vi "Filter Aliases.vi"(8 "error in (no error)":errorcluster, 9 "INI.Client.Type":T1, 10 "Alias.FolderPath":string, 11 "Aliases":string[](array[string])) -> (0 "error out":errorcluster, 2 "Tag.Names":string[](array[string]), 3 "Aliases":string[](array[string]))   [LabVIEW 2019, in "Data Publishing Service.lvlib"]
uses:
  Data Publishing Service.lvlib
  Types/ClientType.ctl
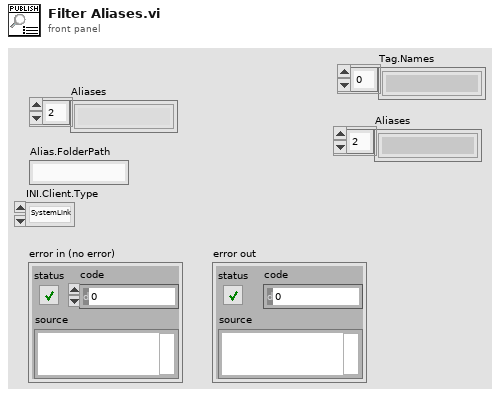
[diagram p1: front panel]
types:
  T1 = typedef "Data Publishing Service.lvlib/ClientType.ctl" = enum16{"SystemLink", "DSC"}
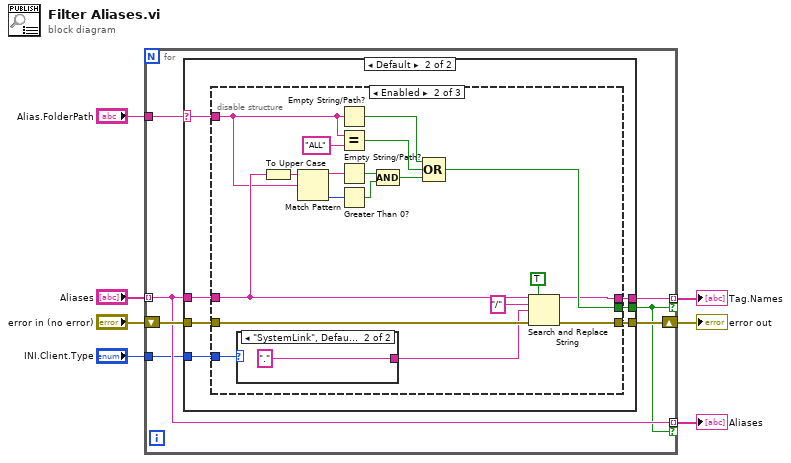
[diagram p0: block diagram]
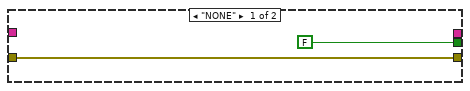
[diagram p2: hidden frame]
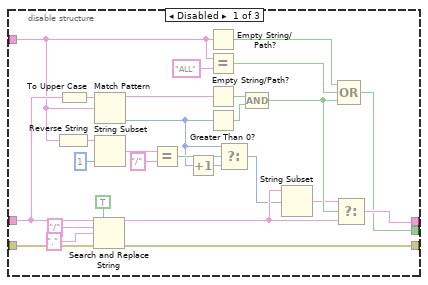
[diagram p3: hidden frame]
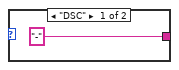
[diagram p4: hidden frame]
diagram:
  n1 = for {
    shift-right: [w13] -> w4
    shift-left: "error in (no error)" -> [w14]
    tunnel: "Aliases" -> [w10] mode=indexing
    tunnel: [w12] -> w3 mode=indexing if=w9
    tunnel: "Alias.FolderPath" -> [w11]
    tunnel: [w10] -> w2 mode=indexing if=w9
    tunnel: "INI.Client.Type" -> [w8]
    n2 = case shown="Default" w11 {
      selector: w11 -> [_ w18]
      tunnel: w14 -> [w16 w21]
      tunnel: w10 -> [_ w20]
      tunnel: [w16 w23] -> w13
      tunnel: [_ w22] -> w12
      tunnel: [FALSE w19] -> w9
      tunnel: w8 -> [_ w17]
      frame "NONE" {
      }
      frame Default {
        n3 = disable-structure shown="Enabled" {
          disable-tunnel: [w50 w69 _] -> w23
          disable-tunnel: [w49 w52 _] -> w22
          disable-tunnel: w21 -> [w41 w61 _]
          disable-tunnel: w20 -> [w39 w59 _]
          disable-tunnel: [w33 w55 _] -> w19
          disable-tunnel: w18 -> [w24 w53 _]
          disable-tunnel: w17 -> [_ w51 _]
          frame Disabled {
            n4 = Reverse String(1:w24) -> (0:w31:string)
            n5 = To Upper Case(1:w39) -> (0:w42:string)
            n6 = Search and Replace String(replace all?=TRUE ("replace all? (F)"), input string=w39, search string="/", replace string="." ("replace string (\"\")"), error in=w41) -> (result string=w35:string, error out=w50:errorcluster)  [unwired: 3 in, 2 out]
            n7 = Match Pattern(string=w42, regular expression=w24) -> (before substring=w46:string, offset past match=w26:i32)  [unwired: 1 in, 2 out]
            n8 = String Subset(string=w31, length (rest)=1 ("length (rest)")) -> (substring=w30:string)  [unwired: 1 in]
            n9 = Equal?(x=w30, y="/" ("search string")) -> (x = y?=w28:bool)
            n10 = Increment(x=w26) -> (x+1=w27:i32)
            n11 = Empty String/Path?(string/path=w24) -> (empty?=w43:bool)
            n12 = Equal?(x=w24, y="ALL" ("x")) -> (x = y?=w47:bool)
            n13 = Empty String/Path?(string/path=w46) -> (empty?=w45:bool)
            n14 = Greater Than 0?(x=w26) -> (x > 0?=w44:bool)
            n15 = Select(t=w26, s=w28, f=w27) -> (s? t:f=w25:i32)
            n16 = Compound Arithmetic op=AND(w45, w44) -> (w36:bool)
            n17 = String Subset(string=w35, offset (0)=w25) -> (substring=w34:string)  [unwired: 1 in]
            n18 = Select(t=w34, s=w36, f=w35) -> (s? t:f=w49:string)
            n19 = Compound Arithmetic op=OR(w43, w47, w36) -> (w33:bool)
          }
          frame Enabled {
            n20 = case shown="\"SystemLink\", Default" w51 {
              tunnel: ["-" ("replace string (\"\")") "." ("replace string (\"\")")] -> w57
              frame "DSC" {
              }
              frame "SystemLink", Default {
              }
            }
            n21 = To Upper Case(1:w59) -> (0:w62:string)
            n22 = Match Pattern(string=w62, regular expression=w53) -> (before substring=w66:string, offset past match=w54:i32)  [unwired: 1 in, 2 out]
            n23 = Empty String/Path?(string/path=w53) -> (empty?=w63:bool)
            n24 = Equal?(x=w53, y="ALL" ("x")) -> (x = y?=w67:bool)
            n25 = Empty String/Path?(string/path=w66) -> (empty?=w65:bool)
            n26 = Greater Than 0?(x=w54) -> (x > 0?=w64:bool)
            n27 = Compound Arithmetic op=AND(w65, w64) -> (w56:bool)
            n28 = Compound Arithmetic op=OR(w63, w67, w56) -> (w55:bool)
            n29 = Search and Replace String(replace all?=TRUE ("replace all? (F)"), input string=w59, search string="/", replace string=w57, error in=w61) -> (result string=w52:string, error out=w69:errorcluster)  [unwired: 3 in, 2 out]
          }
          frame Disabled {
          }
        }
      }
    }
  }
  "error out" <- w4
  "Tag.Names" <- w3
  "Aliases" <- w2
